vi "Init.vi"(4 "Replace":string, 6 "Search":string, 8 "error in (no error)":errorcluster, 9 "RegEx search [T]":bool=TRUE, 10 "Replace all? [F]":bool) -> (0 "error out":errorcluster, 3 "Find First Query out":refnum<class "Search Replace Query.lvclass">)   [LabVIEW 2013, in "Search Replace Query.lvclass"]
doc: "Copyright 2018, Carya Automatisering, Wiebe Walstra."
uses:
  Search Replace Query.lvclass
  Data.ctl
  Search Replace Query.lvclass/Search Replace Query.ctl
  CConfig Object.lvclass
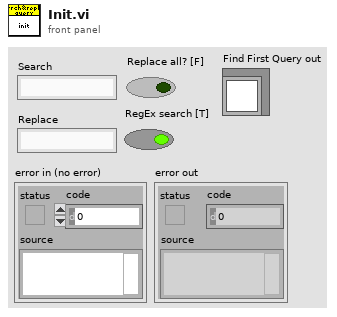
[diagram p1: front panel]
types:
  T1 = typedef "CConfig Object.lvclass/Data.ctl" = enum16{"pre", "name", "middle", "value", "post", "newline", "persistant", "tagged", "type"}
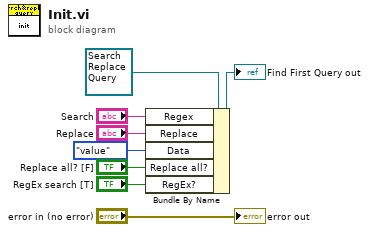
[diagram p0: block diagram]
diagram:
  n1 = Bundle By Name(cluster=refnum<class "Search Replace Query.lvclass"> refnum ("Find First Query in"), "Regex"="Search", "Replace"="Replace", "Data"=Data."value" ("Data [value]"), "Replace all?"="Replace all? [F]", "RegEx?"="RegEx search [T]") -> (→"Find First Query out":refnum<class "Search Replace Query.lvclass">)
  "error out" <- "error in (no error)"
